vi "生成序列值.vi"(10 "改变量":dbl min=0.0, 11 "分段":dbl[](array[numeric])) -> (3 "序列值":dbl[](array[numeric]))   [LabVIEW 2020]
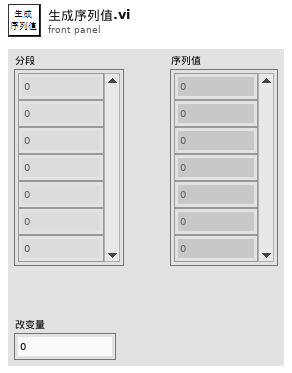
[diagram p1: front panel]
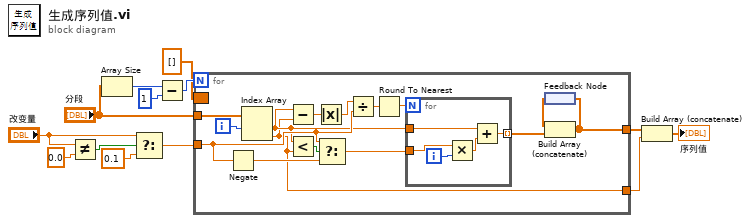
[diagram p0: block diagram]
diagram:
  n1 = Not Equal?(x="改变量", y=0.0 ("x")) -> (x != y?=w8:bool)
  n2 = Array Size(array="分段") -> (size(s)=w13:i32)
  n3 = Select(t="改变量", s=w8, f=0.1) -> (s? t:f=w7:dbl)
  n4 = Subtract(x=w13, y=1) -> (x-y=w11:i32)
  n5 = for {
    N: w11 -> [_]
    tunnel: "分段" -> [w28]
    tunnel: w7 -> [w22]
    border: dbl[] [] -> [_]
    tunnel: [w16] -> w2
    tunnel: [w14] -> w3
    i -> [w27]
    n6 = Negate(x=w22) -> (-x=w21:dbl)
    n7 = Index Array(array=w28, index #1=w27) -> (element #1=w15:dbl, element #2=w14:dbl)  [unwired: 1 in]
    n8 = Subtract(x=w15, y=w14) -> (x-y=w26:dbl)
    n9 = Less?(x=w15, y=w14) -> (x < y?=w20:bool)
    n10 = Absolute Value(x=w26) -> (abs(x)=w25:dbl)
    n11 = Select(t=w22, s=w20, f=w21) -> (s? t:f=w19:dbl)
    n12 = Divide(x=w25, y=w22) -> (x/y=w24:dbl)
    n13 = Round To Nearest(number=w24) -> (nearest integer value=w23:dbl)
    n14 = for {
      N: w23 -> [_]
      tunnel: w19 -> [w31]
      tunnel: [w33] -> w18 mode=indexing
      tunnel: w15 -> [w32]
      i -> [w30]
      n15 = Multiply(x=w31, y=w30) -> (x*y=w29:dbl)
      n16 = Add(x=w32, y=w29) -> (x+y=w33:dbl)
    }
    n17 = feedback #1() -> (w17:dbl[])
    n18 = Build Array (concatenate)(w17, w18) -> (w16:dbl[])
    n19 = feedback-in #1(w16) -> ()
  }
  n20 = Build Array (concatenate)(w2, w3) -> (→"序列值":dbl[])
